vi "Save Project.vi"(8 "Error In":errorcluster, 11 "Proejct In":path) -> (0 "Error Out":errorcluster, 3 "Project Out":path)   [LabVIEW 2017, in "Scripts.lvlib"]
doc: "Saves the project file. During building and packaging of a distribution, the project file may be modified. This leaves unsaved changes and causes a prompt to appear that must save or ignore the modifications before the package \"script\" completes. The prompt blocks execution, so inclusion in an automated build is difficult. This VI saves the project and avoids the prompt."
uses:
  Scripts.lvlib
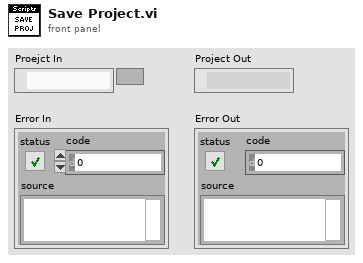
[diagram p1: front panel]
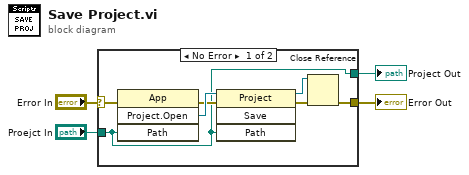
[diagram p0: block diagram]
diagram:
  n1 = case shown="No Error" "Error In" {
    selector: "Error In" -> [w6 w13]
    tunnel: [w10 w13] -> w4
    tunnel: "Proejct In" -> [w5 w12]
    tunnel: [w5 w12] -> w1
    frame No Error {
      n2 = invoke class="App" method="Project.Open"(error in=w6, "Path"=w5) -> (error out=w7:errorcluster, "Project:Open"=w9:refnum<vi>)  [unwired: 2 in, 2 out]
      n3 = invoke class="Project" method="Save"(reference=w9, error in=w7, "Path"=w5) -> (reference out=w11:refnum<vi>, error out=w8:errorcluster)  [unwired: 1 in, 2 out]
      n4 = Close Reference(reference=w11, error in (no error)=w8) -> (error out=w10:errorcluster)
    }
    frame Error {
    }
  }
  "Error Out" <- w4
  "Project Out" <- w1
